vi "GetSlopeConductance.vi"(11 "Array in":dbl[][](array[numeric])) -> (2 "Fit":dbl[](array[numeric]))   [LabVIEW 2020]
uses:
  <vilib>/Analysis/6fits.llb/Curve Fitting Criteria.ctl
  <vilib>/Analysis/NI_AALPro.lvlib
panel:
  out "XY Graph":cluster{dbl[], dbl[]}[](graph)
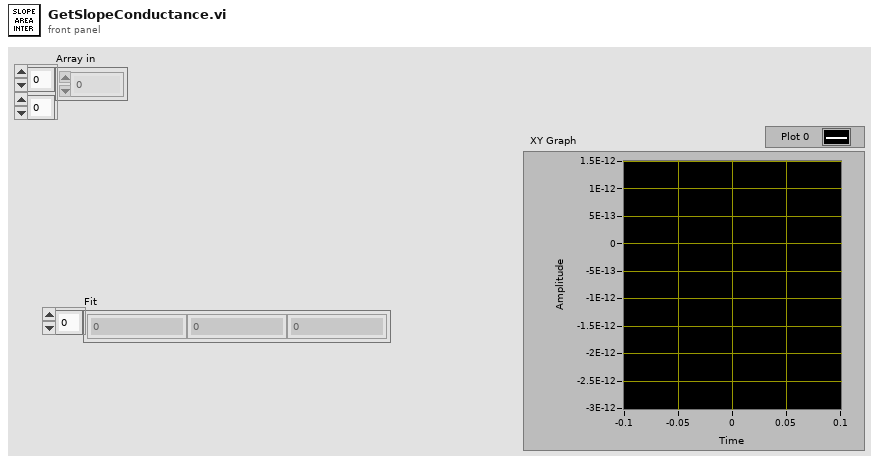
[diagram p1: front panel]
types:
  T1 = typedef "NI_AALPro.lvlib/Curve Fitting Criteria.ctl" = u16
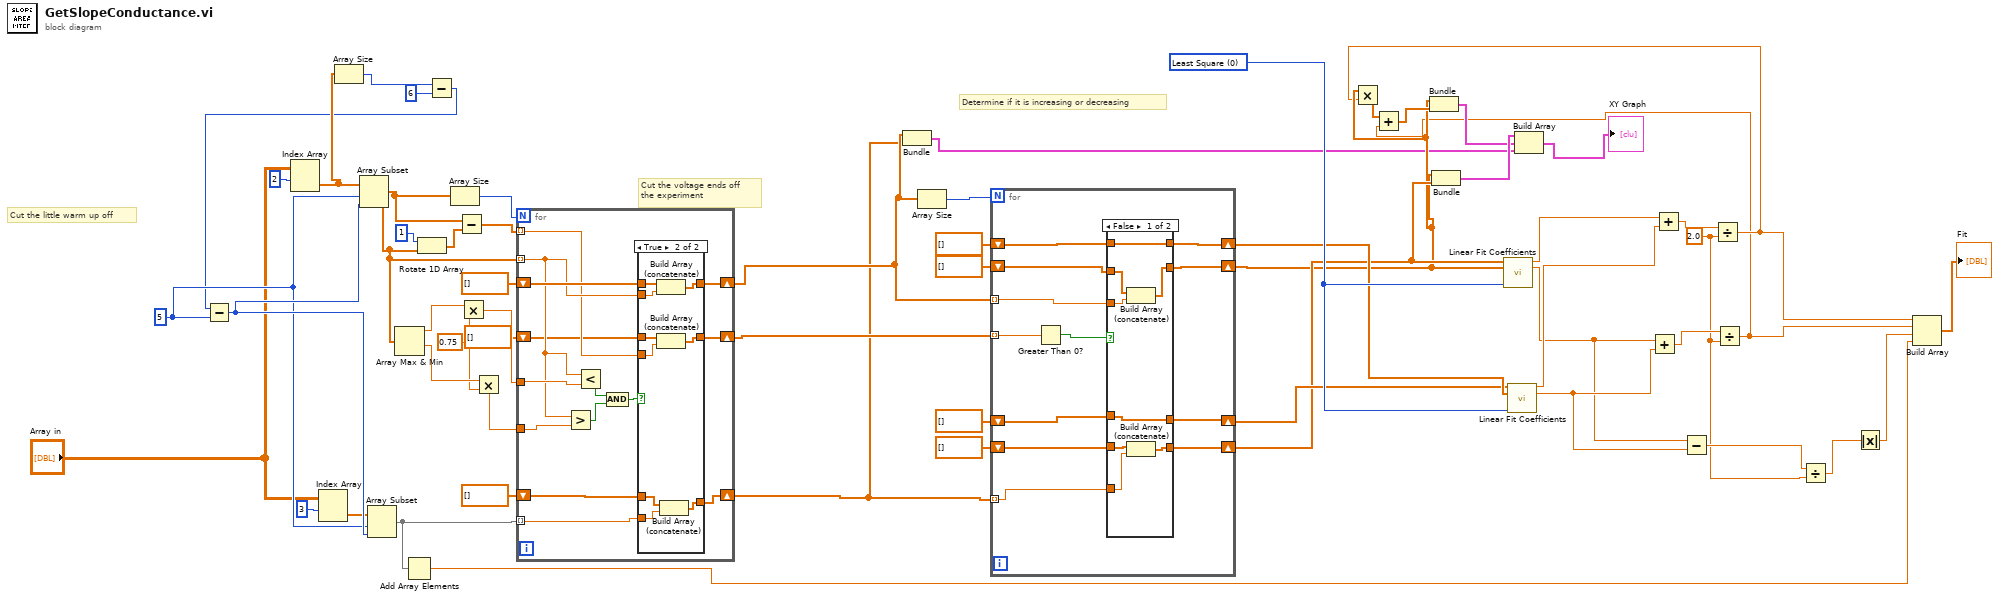
[diagram p0: block diagram]
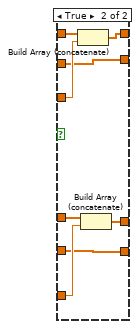
[diagram p2: hidden frame]
diagram:
  w30 = 2.0 ("y")
  w50 = 0.75 ("y")
  w56 = 5 ("y")
  w45 = T1 0 items=["Least Square", "Least Absolute Residual", "Bisquare"] ("method")
  # "Determine if it is increasing or decreasing"
  # "Cut the little warm up off"
  # "Cut the voltage ends off\nthe experiment"
  n1 = Index Array(array="Array in", index (row)=2) -> (element=w26:dbl[])  [unwired: 1 in]
  n2 = Index Array(array="Array in", index (row)=3) -> (element=w53:dbl[])  [unwired: 1 in]
  n3 = Array Size(array=w26) -> (size(s)=w25:i32)
  n4 = Subtract(x=w25, y=6) -> (x-y=w23:i32)
  n5 = Subtract(x=w23, y=w56) -> (x-y=w57:i32)
  n6 = Array Subset(array=w26, index=w56, length=w57) -> (w41:dbl[])
  n7 = Array Subset(array=w53, index=w56, length=w57) -> (w44:dbl[])
  n8 = Array Max & Min(array=w41) -> (max value=w52:dbl, min value=w51:dbl)  [unwired: 2 out]
  n9 = Add Array Elements(numeric array=w44) -> (sum=w27:dbl)
  n10 = Rotate 1D Array(1:w41, 2:1 ("n")) -> (0:w42:dbl[])
  n11 = Array Size(array=w41) -> (size(s)=w49:i32)
  n12 = Subtract(x=w41, y=w42) -> (x-y=w40:dbl[])
  n13 = Multiply(x=w52, y=w50) -> (x*y=w48:dbl)
  n14 = Multiply(x=w51, y=w50) -> (x*y=w47:dbl)
  n15 = for {
    N: w49 -> [_]
    tunnel: w41 -> [w64] mode=indexing
    tunnel: w44 -> [w63] mode=indexing
    tunnel: w48 -> [w68]
    tunnel: w47 -> [w67]
    shift-right: [w65] -> w5
    shift-left: dbl[] [] -> [w66]
    shift-right: [w62] -> w4
    shift-left: dbl[] [] -> [w61]
    tunnel: w40 -> [w60] mode=indexing
    shift-right: [w59] -> w39
    shift-left: dbl[] [] -> [w58]
    n16 = Greater?(x=w64, y=w67) -> (0:w69:bool)
    n17 = Less?(x=w64, y=w68) -> (x < y?=w71:bool)
    n18 = And(x=w71, y=w69) -> (x .and. y?=w70:bool)
    n19 = case shown="True" w70 {
      tunnel: w66 -> [w74 w82]
      tunnel: [w74 w83] -> w65
      tunnel: w64 -> [_ w81]
      tunnel: w63 -> [_ w80]
      tunnel: [w73 w79] -> w62
      tunnel: w61 -> [w73 w78]
      tunnel: w60 -> [_ w77]
      tunnel: [w72 w76] -> w59
      tunnel: w58 -> [w72 w75]
      frame False {
      }
      frame True {
        n20 = Build Array (concatenate)(w82, w81) -> (w83:dbl[])
        n21 = Build Array (concatenate)(w75, w77) -> (w76:dbl[])
        n22 = Build Array (concatenate)(w78, w80) -> (w79:dbl[])
      }
    }
  }
  n23 = Bundle(w5, w4) -> (w3:cluster{dbl[], dbl[]})  [unwired: 1 in]
  n24 = Array Size(array=w5) -> (size(s)=w46:i32)
  n25 = for {
    N: w46 -> [_]
    tunnel: w5 -> [w93] mode=indexing
    tunnel: w39 -> [w92] mode=indexing
    shift-right: [w94] -> w38
    shift-left: dbl[] [] -> [w95]
    shift-right: [w84] -> w8
    shift-left: dbl[] [] -> [w85]
    shift-right: [w86] -> w37
    shift-left: dbl[] [] -> [w87]
    shift-right: [w90] -> w11
    shift-left: dbl[] [] -> [w89]
    tunnel: w4 -> [w88] mode=indexing
    n26 = Greater Than 0?(x=w92) -> (x > 0?=w91:bool)
    n27 = case shown="False" w91 {
      tunnel: w95 -> [w103 w110]
      tunnel: [w103 w111] -> w94
      tunnel: w93 -> [w98 w109]
      tunnel: w88 -> [w97 w108]
      tunnel: [w102 w104] -> w84
      tunnel: [w101 w107] -> w90
      tunnel: w89 -> [w99 w107]
      tunnel: w85 -> [w100 w104]
      tunnel: w87 -> [w96 w106]
      tunnel: [w96 w105] -> w86
      frame False {
        n28 = Build Array (concatenate)(w100, w98) -> (w102:dbl[])
        n29 = Build Array (concatenate)(w99, w97) -> (w101:dbl[])
      }
      frame True {
        n30 = Build Array (concatenate)(w110, w109) -> (w111:dbl[])
        n31 = Build Array (concatenate)(w106, w108) -> (w105:dbl[])
      }
    }
  }
  n32 = Bundle(w8, w11) -> (w14:cluster{dbl[], dbl[]})  [unwired: 1 in]
  n33 = call <vilib>:"Linear Fit Coefficients.vi"("Y"=w11, "X"=w8, "method"=w45) -> ("slope"=w7:dbl, "intercept"=w6:dbl)  [unwired: 10 in, 1 out]
  n34 = call <vilib>:"Linear Fit Coefficients.vi"("Y"=w37, "X"=w38, "method"=w45) -> ("slope"=w36:dbl, "intercept"=w32:dbl)  [unwired: 10 in, 1 out]
  n35 = Add(x=w6, y=w32) -> (x+y=w34:dbl)
  n36 = Add(x=w7, y=w36) -> (x+y=w35:dbl)
  n37 = Subtract(x=w6, y=w32) -> (x-y=w31:dbl)
  n38 = Divide(x=w35, y=w30) -> (x/y=w2:dbl)
  n39 = Multiply(x=w8, y=w2) -> (x*y=w10:dbl[])
  n40 = Divide(x=w34, y=w30) -> (x/y=w1:dbl)
  n41 = Add(x=w10, y=w1) -> (x+y=w9:dbl[])
  n42 = Bundle(w8, w9) -> (w13:cluster{dbl[], dbl[]})  [unwired: 1 in]
  n43 = Build Array(w14, w13, w3) -> (→"XY Graph":cluster{dbl[], dbl[]}[])
  n44 = Divide(x=w31, y=w30) -> (x/y=w29:dbl)
  n45 = Absolute Value(x=w29) -> (abs(x)=w28:dbl)
  n46 = Build Array(w2, w1, w28, w27) -> (→"Fit":dbl[])
